vi "Query (CryoCon_one time).vi"(2 "error in (no error)":errorcluster, 3 "write buffer":string, 4 "byte count":u32, 5 "VISA resource name 2":refnum<visa-resource-name>) -> (0 "error out":errorcluster, 1 "read buffer":string)   [LabVIEW 2011]
uses:
  <vilib>/Instr/_visa.llb/VISA Configure Serial Port (Instr).vi
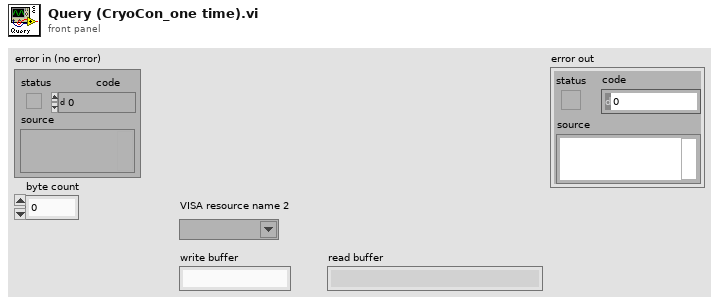
[diagram p1: front panel]
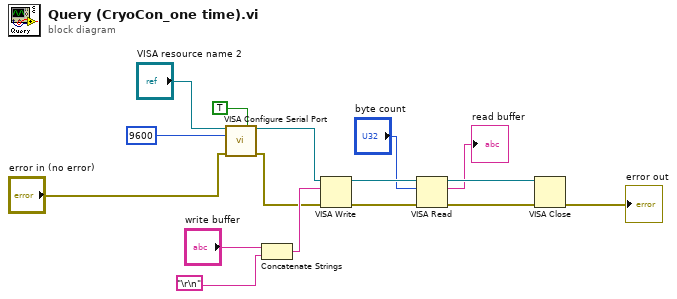
[diagram p0: block diagram]
diagram:
  n1 = call-poly "VISA Configure Serial Port"("VISA resource name"="VISA resource name 2", "Enable Termination\nChar (T)"=TRUE ("Enable Termination\nChar (T)"), "baud rate (9600)"=u32 9600, "error in (no error)"="error in (no error)") -> ("VISA resource name out"=w9:refnum<visa-resource-name>, "error out"=w10:errorcluster)  [unwired: 10 in]
  n2 = Concatenate Strings("write buffer", "\r\n") -> (w14:string)
  n3 = VISA Write(VISA resource name=w9, write buffer=w14, error in (no error)=w10) -> (VISA resource name out=w16:refnum<visa-resource-name>, error out=w7:errorcluster)  [unwired: 1 out]
  n4 = VISA Read(VISA resource name=w16, byte count="byte count", error in (no error)=w7) -> (VISA resource name out=w5:refnum<visa-resource-name>, read buffer=→"read buffer":string, error out=w6:errorcluster)  [unwired: 1 out]
  n5 = VISA Close(VISA resource name=w5, error in (no error)=w6) -> (error out=→"error out":errorcluster)
